vi "Remove Client Handler.vi"(8 "error in (no error)":errorcluster, 10 "GUID":string, 11 "Websocket Server in":refnum<class "Websocket Server.lvclass">) -> (0 "error out":errorcluster, 3 "Websocket Server out":refnum<class "Websocket Server.lvclass">)   [LabVIEW 2016, in "Stream Mediator.lvlib" / "Websocket Server.lvclass"]
uses:
  <userlib>/Composed Systems/Stream/Mediator/Classes/Websocket Server Actor/Websocket Server/Websocket Server.lvclass
  <userlib>/Composed Systems/Stream/Mediator/Classes/Websocket Server Actor/Websocket Server/Websocket Server.lvclass/Websocket Server.ctl
  <userlib>/Composed Systems/Stream/Mediator/Classes/Subscriber Look Up Table/Subscriber Look Up Table.lvclass
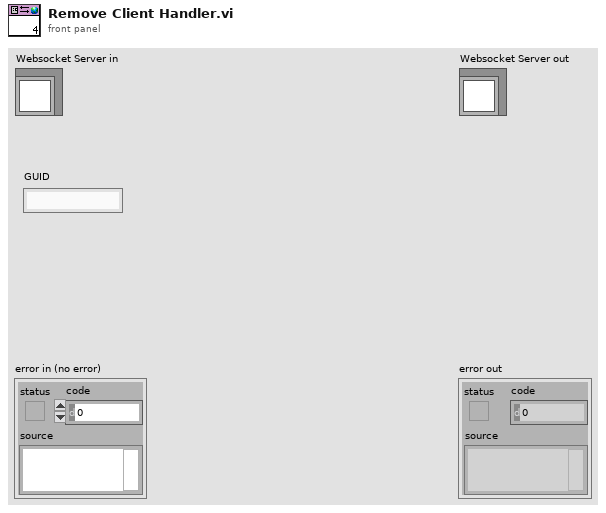
[diagram p1: front panel]
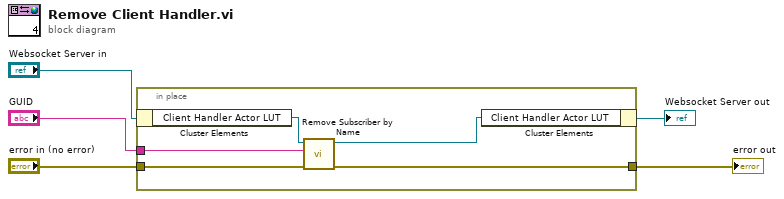
[diagram p0: block diagram]
diagram:
  n1 = in-place {
    in-place-border: "GUID" -> [w8]
    in-place-border: "error in (no error)" -> [w9]
    in-place-border: [w6] -> w1
    n2 = in-place-cluster #1("Websocket Server in") -> ("Client Handler Actor LUT"=w10:refnum<class "Subscriber Look Up Table.lvclass">)
    n3 = call <userlib>:"Remove Subscriber by Name.vi"("error in (no error)"=w9, "Topic Name"=w8, "Subscriber Look Up Table in"=w10) -> ("error out"=w6:errorcluster, "Subscriber Look Up Table out"=w7:refnum<class "Subscriber Look Up Table.lvclass">)  [unwired: 6 in, 1 out]
    n4 = in-place-cluster #1("Client Handler Actor LUT"=w7) -> (→"Websocket Server out":refnum<class "Websocket Server.lvclass">)
  }
  "error out" <- w1
